vi "Apply Button Dialog Parameters.vi"(0 "Indicator left position":dbl, 1 "Max Message Indicator Width":dbl, 2 "Min Message Indicator Width":dbl, 3 "Max Message Indicator Height":dbl, 5 "Calculated indicator height":dbl, 7 "Indicator height scaled large":dbl, 9 "Actual indicator height":dbl, 11 "Indicator height scaled small":dbl, 12 "right":i16) -> (4 "Message indicator size":T1, 6 "Message indicator left":i32, 8 "Message indicator top":i32, 10 "VScrolVis":bool, 14 "Panel origin vertical":i16, 15 "Panel bounds top":i16)   [LabVIEW 2010]
uses:
  <vilib>/Utility/miscctls.llb/LVBoundsTypeDef.ctl
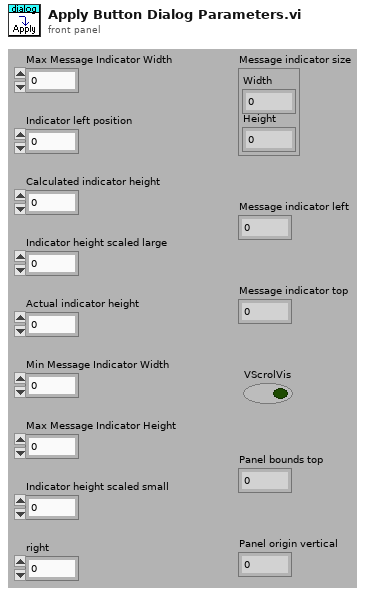
[diagram p1: front panel]
types:
  T1 = typedef "LVBoundsTypeDef.ctl" = cluster{"Width":u32, "Height":u32}
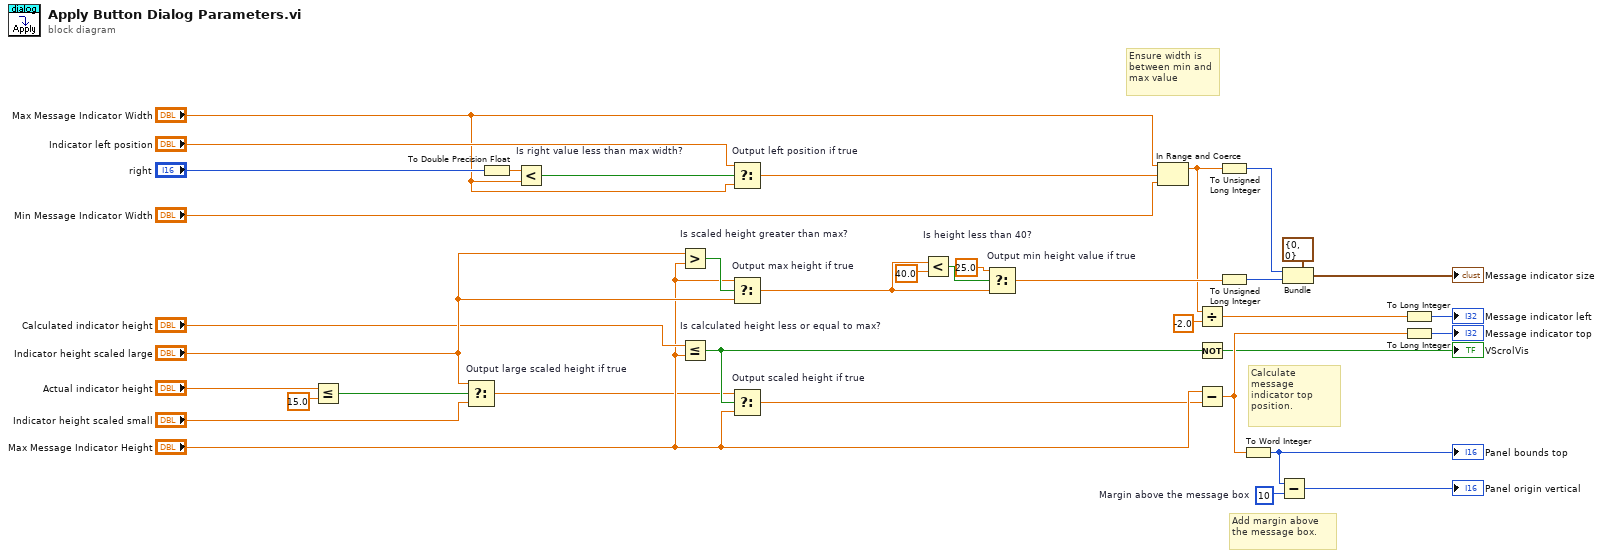
[diagram p0: block diagram]
diagram:
  w14 = i16 10  # Margin above the message box
  # "Ensure width is between min and max value"
  # "Add margin above the message box."
  # "Calculate message indicator top position."
  n1 = Less Or Equal?(x="Actual indicator height", y=15.0) -> (x <= y?=w9:bool)
  n2 = Select "Output large scaled height if true"(t="Indicator height scaled large", s=w9, f="Indicator height scaled small") -> (s? t:f=w10:dbl)
  n3 = To Double Precision Float(number="right") -> (double precision float=w24:dbl)
  n4 = Less? "Is right value less than max width?"(x=w24, y="Max Message Indicator Width") -> (x < y?=w5:bool)
  n5 = Greater? "Is scaled height greater than max?"(x="Indicator height scaled large", y="Max Message Indicator Height") -> (0:w34:bool)
  n6 = Less Or Equal? "Is calculated height less or equal to max?"(x="Calculated indicator height", y="Max Message Indicator Height") -> (x <= y?=w22:bool)
  n7 = Select "Output left position if true"(t="Indicator left position", s=w5, f="Max Message Indicator Width") -> (s? t:f=w13:dbl)
  n8 = Select "Output max height if true"(t="Max Message Indicator Height", s=w34, f="Indicator height scaled large") -> (s? t:f=w17:dbl)
  n9 = Select "Output scaled height if true"(t=w10, s=w22, f="Max Message Indicator Height") -> (s? t:f=w20:dbl)
  n10 = Less? "Is height less than 40?"(x=w17, y=40.0) -> (x < y?=w16:bool)
  n11 = Select "Output min height value if true"(t=25.0, s=w16, f=w17) -> (s? t:f=w18:dbl)
  n12 = In Range and Coerce(upper limit="Max Message Indicator Width", x=w13, lower limit="Min Message Indicator Width") -> (coerced(x)=w1:dbl)  [unwired: 1 out]
  n13 = Divide(x=w1, y=-2.0) -> (x/y=w21:dbl)
  n14 = Not(x=w22) -> (.not. x?=→"VScrolVis":bool)
  n15 = Subtract(x="Max Message Indicator Height", y=w20) -> (x-y=w35:dbl)
  n16 = To Unsigned Long Integer(number=w1) -> (unsigned 32bit integer=w25:u32)
  n17 = To Unsigned Long Integer(number=w18) -> (unsigned 32bit integer=w26:u32)
  n18 = To Word Integer(number=w35) -> (16bit integer=w36:i16)
  "Panel bounds top" <- w36
  n19 = Subtract(x=w36, y=w14) -> (x-y=→"Panel origin vertical":i16)
  n20 = Bundle(cluster=T1 {"Width"=0, "Height"=0} ("Size"), "Width"=w25, "Height"=w26) -> (→"Message indicator size":T1)
  n21 = To Long Integer(number=w21) -> (32bit integer=→"Message indicator left":i32)
  n22 = To Long Integer(number=w35) -> (32bit integer=→"Message indicator top":i32)
